vi "ShiftRegisters.vi"() -> ()   [LabVIEW 2014]
panel:
  in  "N terms":i32=10
  in  "y0 and y1":dbl[](array[numeric])=[0.0, 1.0]
  out "Y":dbl[](array[numeric])
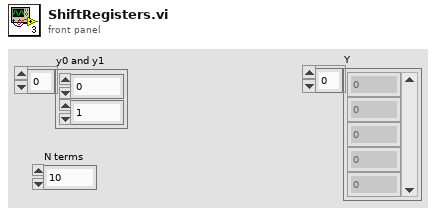
[diagram p1: front panel]
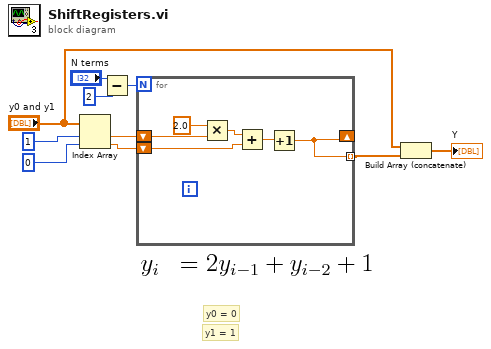
[diagram p0: block diagram]
diagram:
  # "y1 = 1"
  # "y0 = 0"
  n1 = Index Array(array="y0 and y1", index #1=1 ("index"), index #2=0 ("index")) -> (element #1=w3:dbl, element #2=w2:dbl)
  n2 = Subtract(x="N terms", y=2) -> (x-y=w6:i32)
  n3 = for {
    N: w6 -> [_]
    shift-right: [w11] -> _
    shift-left: w3 -> [w16]
    shift-left: w2 -> [w13]
    tunnel: [w11] -> w1 mode=indexing
    n4 = Multiply(x=2.0, y=w16) -> (x*y=w14:dbl)
    n5 = Add(x=w14, y=w13) -> (x+y=w12:dbl)
    n6 = Increment(x=w12) -> (x+1=w11:dbl)
  }
  n7 = Build Array (concatenate)("y0 and y1", w1) -> (→"Y":dbl[])
